vi "VolumeScanWizard 2.0.vi"(10 "Device order":i32[](array[numeric])=[0, 1], 11 "Device description":string[][](array[string])) -> (3 "Output":dbl[][](array[numeric]))   [LabVIEW 2015]
uses:
  <vilib>/gmath/NI_Gmath.lvlib
panel:
  in  "Cancel Button":bool
  in  "OK Button":bool
  in  "Ordering":u16(ring) items=["Raster", "Serpentine"]
  in  "Expression":string
  in  "Scan pattern":u16(ring) items=["Linear", "Exponential", "Logarithmic", "Quadratic", "Custom"]
  in  "Parameter table":string[][](table)
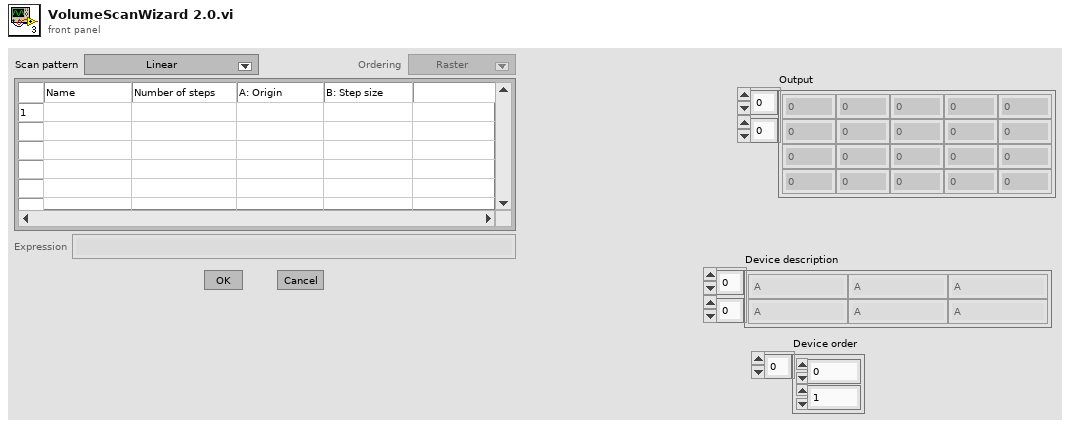
[diagram p1: front panel]
types:
  T1 = enum8{"Enabled", "Disabled", "Disabled and Grayed Out"}
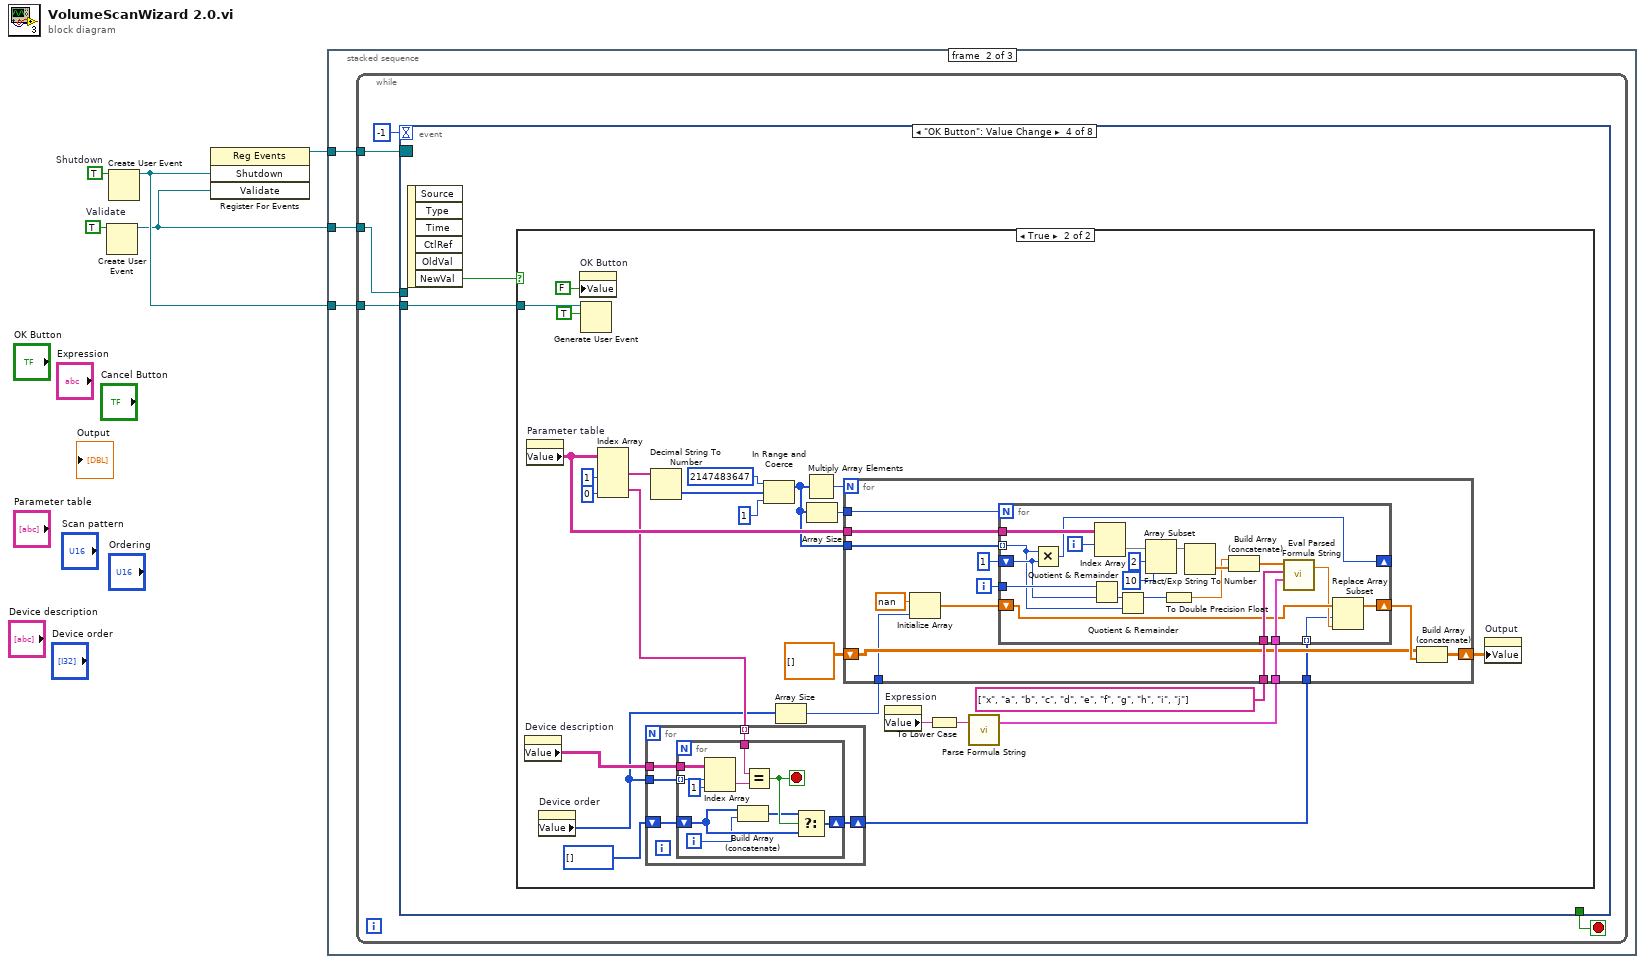
[diagram p0: block diagram]
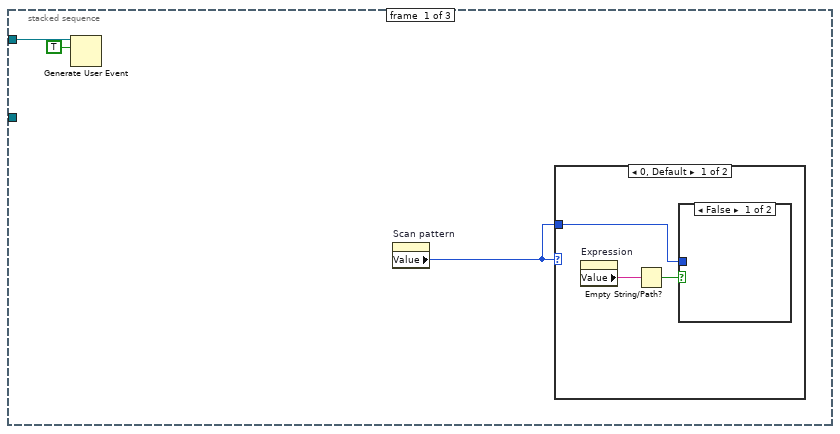
[diagram p2: hidden frame]
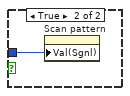
[diagram p3: hidden frame]
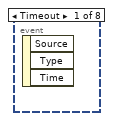
[diagram p5: hidden frame]
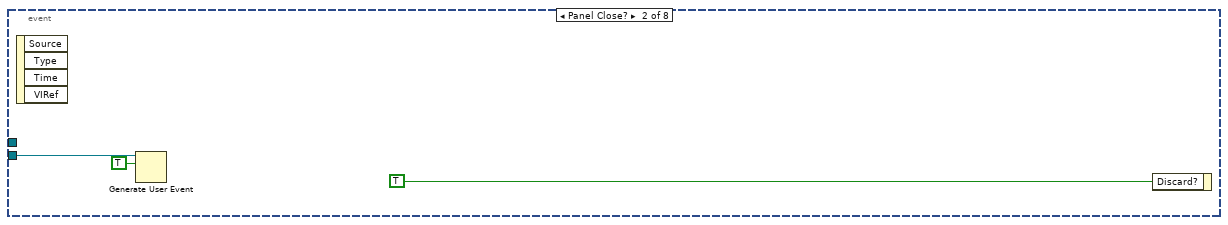
[diagram p6: hidden frame]
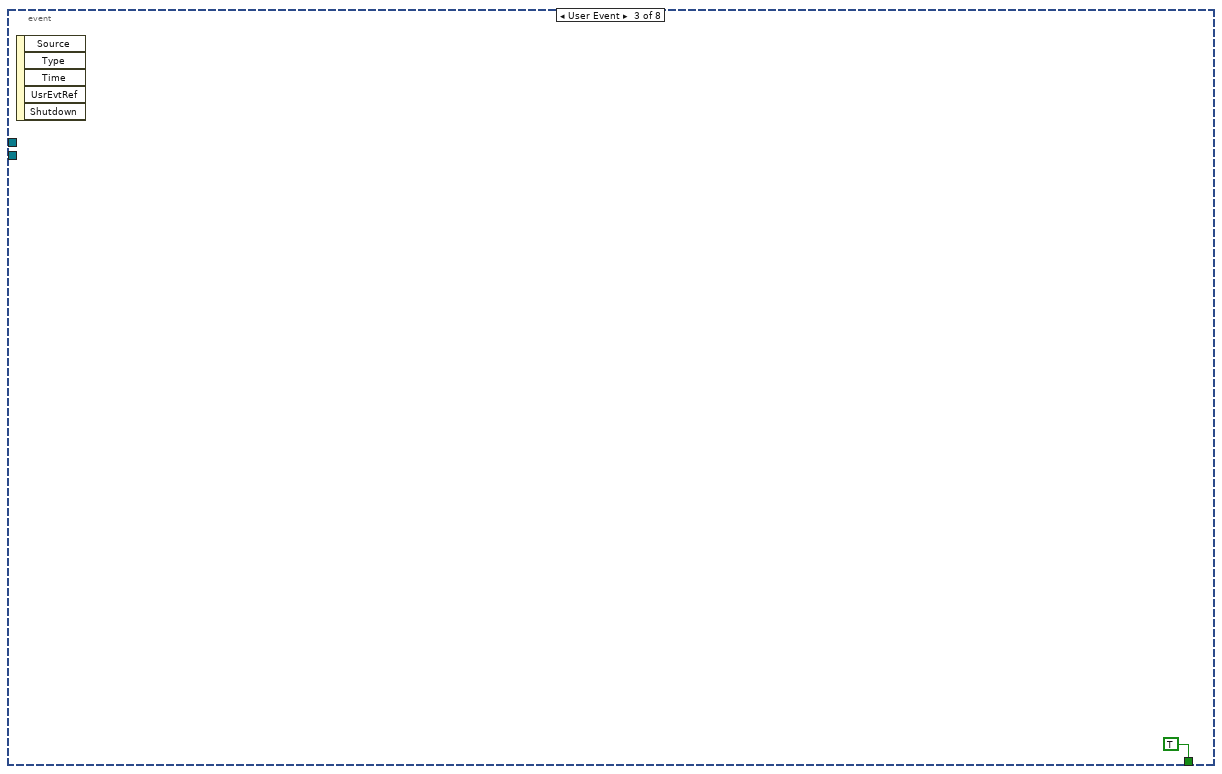
[diagram p7: hidden frame]
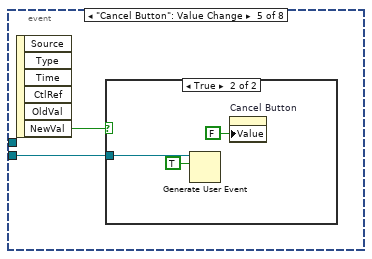
[diagram p9: hidden frame]
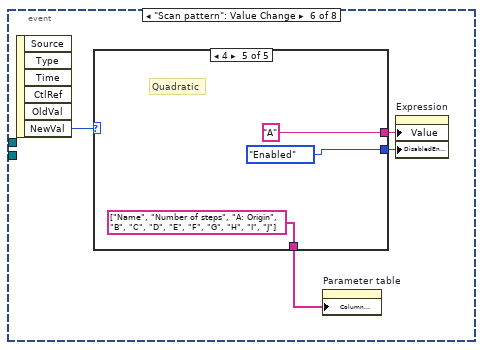
[diagram p11: hidden frame]
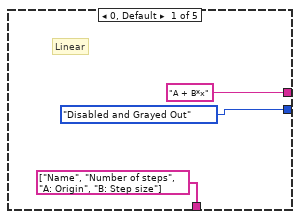
[diagram p12: hidden frame]
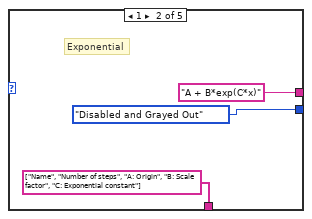
[diagram p13: hidden frame]
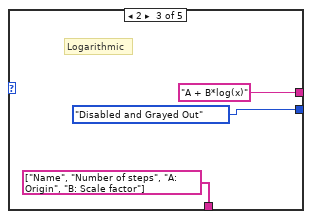
[diagram p14: hidden frame]
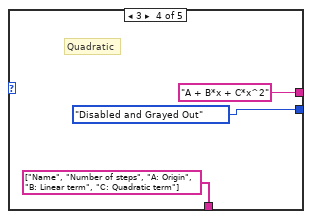
[diagram p15: hidden frame]
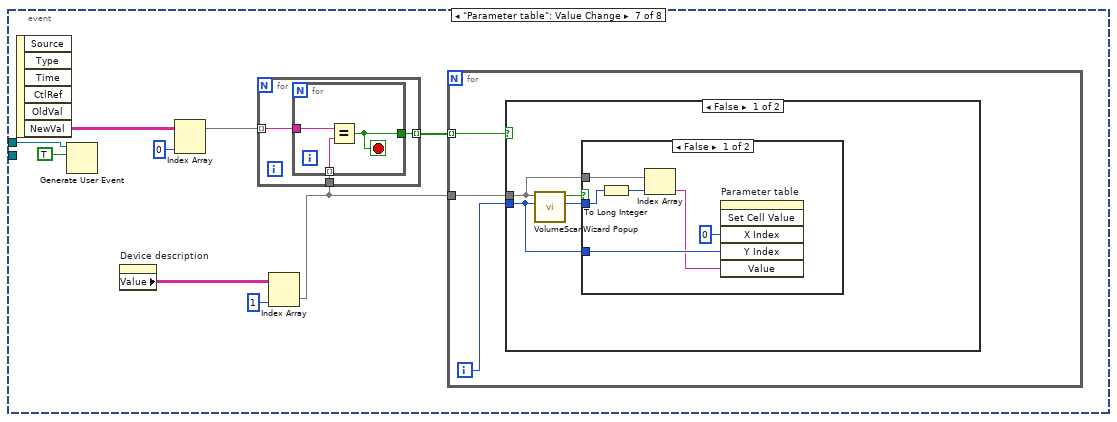
[diagram p16: hidden frame]
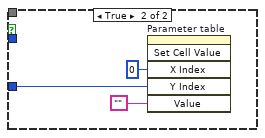
[diagram p17: hidden frame]
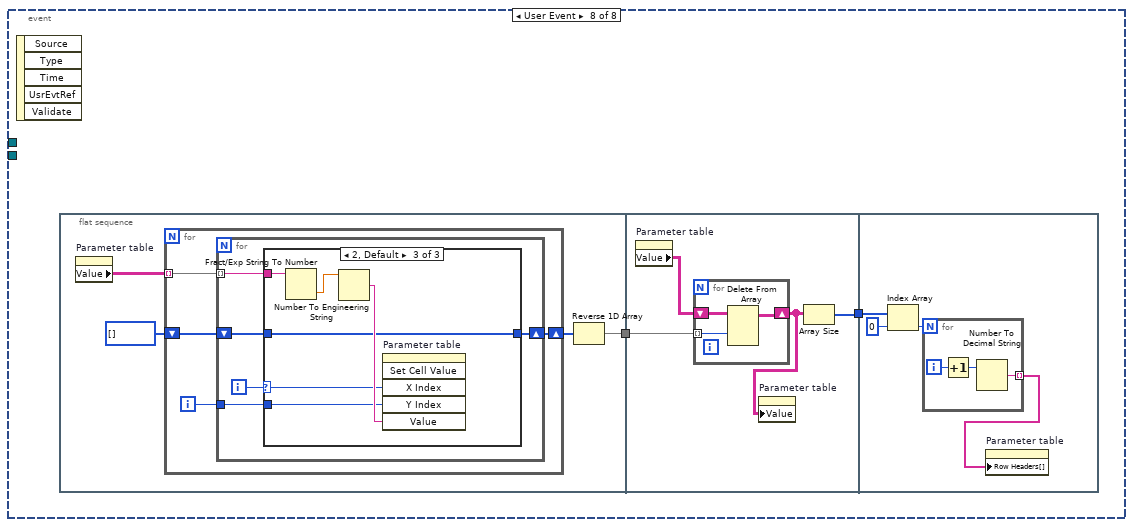
[diagram p19: hidden frame]
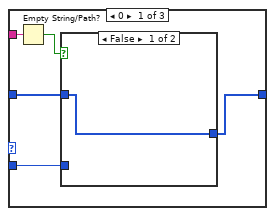
[diagram p20: hidden frame]
diagram:
  w2 = TRUE  # Validate
  w4 = TRUE  # Shutdown
  n1 = Create User Event(user event datatype=w2) -> (user event=w1:refnum<user-event>)  [unwired: 1 in, 1 out]
  n2 = Create User Event(user event datatype=w4) -> (user event=w3:refnum<user-event>)  [unwired: 1 in, 1 out]
  n3 = register-events(w3, w1) -> (reference out=w5:refnum<event-registration>)  [unwired: 2 in, 1 out]
  n4 = stacked-sequence {
    tunnel: w5 -> [_ w15 _]
    tunnel: w3 -> [_ w14 w207]
    tunnel: w1 -> [w8 w13 w208]
    frame #0 {
      n5 = Generate User Event(user event=w8, event data cluster=TRUE ("event data")) -> ()  [unwired: 2 in, 2 out]
      n6 = property on="Scan pattern" class="Ring (strict)"() -> ("Value"=w6:u16)  [unwired: 2 in, 2 out]
      n7 = case shown="0, Default" w6 {
        tunnel: w6 -> [w9 _]
        frame 0, Default {
          n8 = property on="Expression" class="Str"() -> ("Value"=w11:string)  [unwired: 2 in, 2 out]
          n9 = Empty String/Path?(string/path=w11) -> (empty?=w10:bool)
          n10 = case shown="False" w10 {
            tunnel: w9 -> [_ w12]
            frame False {
            }
            frame True {
              n11 = property on="Scan pattern" class="Ring (strict)"("Val(Sgnl)"=w12) -> ()  [unwired: 2 in, 2 out]
            }
          }
        }
        frame 4 {
        }
      }
    }
    frame #1 {
      n12 = while {
        tunnel: w15 -> [w19]
        tunnel: w14 -> [w17]
        tunnel: w13 -> [w16]
        stop <- w18 stop-if-true
        n13 = event shown="[3] \"OK Button\": Value Change" {
          selector: w19 -> [_ _ _ _ _ _ _ _]
          dyn-events: _ -> [_ _ _ _ _ _ _ _]
          timeout: -1 -> [_ _ _ _ _ _ _ _]
          tunnel: [_ _ TRUE _ _ _ _ _] -> w18
          tunnel: w17 -> [_ w22 _ w26 w103 _ _ _]
          tunnel: w16 -> [_ _ _ _ _ _ w134 _]
          event Timeout {
            n14 = event-data() -> ()  [unwired: 1 in, 3 out]
          }
          event Panel Close? {
            n15 = event-data() -> ()  [unwired: 1 in, 4 out]
            n16 = Generate User Event(user event=w22, event data cluster=TRUE ("event data")) -> ()  [unwired: 2 in, 2 out]
            n17 = event-data("Discard?"=TRUE) -> ()  [unwired: 1 in, 1 out]
          }
          event User Event {
            n18 = event-data() -> ()  [unwired: 1 in, 5 out]
          }
          event "OK Button": Value Change {
            n19 = event-data() -> ("NewVal"=w25:bool)  [unwired: 1 in, 5 out]
            n20 = case shown="True" w25 {
              tunnel: w26 -> [_ w51]
              frame False {
              }
              frame True {
                n21 = property on="Device description" class="Arr (strict)"() -> ("Value"=w32:string[][])  [unwired: 2 in, 2 out]
                n22 = property on="Parameter table" class="Tbl (strict)"() -> ("Value"=w41:string[][])  [unwired: 2 in, 2 out]
                n23 = property on="Device order" class="Arr (strict)"() -> ("Value"=w27:i32[])  [unwired: 2 in, 2 out]
                n24 = property on="OK Button" class="Bool (strict)"("Value"=FALSE ("OK Button")) -> ()  [unwired: 2 in, 2 out]
                n25 = Generate User Event(user event=w51, event data cluster=TRUE ("event data")) -> ()  [unwired: 2 in, 2 out]
                n26 = Index Array(array=w41, index (col) #1=1 ("disabled index (col)"), index (col) #2=0 ("index (col)")) -> (element #1=w47:string[], element #2=w31:string[])  [unwired: 2 in]
                n27 = for {
                  tunnel: w32 -> [w56]
                  tunnel: w27 -> [w55]
                  tunnel: w31 -> [w54] mode=indexing
                  shift-right: [w52] -> w29
                  shift-left: i32[] [] -> [w53]
                  n28 = for {
                    tunnel: w56 -> [w66]
                    tunnel: w55 -> [w65] mode=indexing
                    tunnel: w54 -> [w63]
                    shift-right: [w61] -> w52
                    shift-left: w53 -> [w60]
                    i -> [w57]
                    stop <- w62 stop-if-true
                    n29 = Index Array(array=w66, index (row)=w65, index (col)=1 ("disabled index (col)")) -> (element=w58:string)
                    n30 = Build Array (concatenate)(w60, w57) -> (w59:i32[])
                    n31 = Equal?(x=w63, y=w58) -> (x = y?=w62:bool)
                    n32 = Select(t=w59, s=w62, f=w60) -> (s? t:f=w61:i32[])
                  }
                }
                n33 = Decimal String To Number(string=w47) -> (number=w46:i32[])  [unwired: 2 in, 1 out]
                n34 = In Range and Coerce(upper limit=2147483647, x=w46, lower limit=1) -> (coerced(x)=w38:i32[])  [unwired: 1 out]
                n35 = Array Size(array=w27) -> (size(s)=w28:i32)
                n36 = Multiply Array Elements(1:w38) -> (0:w44:i32)
                n37 = Array Size(array=w38) -> (size(s)=w43:i32)
                n38 = property on="Expression" class="Str"() -> ("Value"=w35:string)  [unwired: 2 in, 2 out]
                n39 = To Lower Case(string=w35) -> (all lower case string=w34:string)
                n40 = call <vilib>:"Parse Formula String.vi"("formula"=w34) -> ("Parsed Formula"=w40:cluster{"Table":i32[][], "Y Values":dbl[]})  [unwired: 1 in, 1 out]
                n41 = for {
                  N: w44 -> [_]
                  tunnel: w43 -> [w78]
                  tunnel: w41 -> [w80]
                  tunnel: w40 -> [w76]
                  tunnel: string[] ["x", "a", "b", "c", "d", "e", "f", "g", "h", "i", "j"] ("Variables") -> [w75]
                  tunnel: w38 -> [w70]
                  shift-right: [w71] -> w36
                  shift-left: dbl[][] [] -> [w72]
                  tunnel: w29 -> [w68]
                  tunnel: w28 -> [w67]
                  i -> [w74]
                  n42 = Initialize Array(nan ("element"), w67) -> (w79:dbl[])
                  n43 = for {
                    N: w78 -> [_]
                    tunnel: w80 -> [w101]
                    shift-right: [w89] -> w73
                    shift-left: w79 -> [w88]
                    tunnel: w76 -> [w97]
                    tunnel: w75 -> [w96]
                    tunnel: w74 -> [w85]
                    shift-right: [w92] -> _
                    shift-left: 1 -> [w83]
                    tunnel: w70 -> [w82] mode=indexing
                    tunnel: w68 -> [w81] mode=indexing
                    i -> [w86]
                    n44 = Multiply(x=w82, y=w83) -> (x*y=w92:i32)
                    n45 = Quotient & Remainder(x=w85, y=w83) -> (floor(x/y)=w84:i32)  [unwired: 1 out]
                    n46 = Index Array(array=w101, index (row)=w86) -> (element=w100:string[])  [unwired: 1 in]
                    n47 = Quotient & Remainder(x=w84, y=w82) -> (x-y*floor(x/y)=w91:i32)  [unwired: 1 out]
                    n48 = Array Subset(array=w100, index=2, length=10) -> (w99:string[])
                    n49 = To Double Precision Float(number=w91) -> (double precision float=w90:dbl)
                    n50 = Fract/Exp String To Number(string=w99) -> (number=w95:dbl[])  [unwired: 3 in, 1 out]
                    n51 = Build Array (concatenate)(w90, w95) -> (w94:dbl[])
                    n52 = call <vilib>:"Eval Parsed Formula String.vi"("Parsed Formula"=w97, "Variables"=w96, "X Values"=w94) -> ("y value"=w87:dbl)  [unwired: 1 in, 1 out]
                    n53 = Replace Array Subset(array=w88, new element=w87, index=w81) -> (w89:dbl[])
                  }
                  n54 = Build Array (concatenate)(w72, w73) -> (w71:dbl[][])
                }
                n55 = property on="Output" class="Arr (strict)"("Value"=w36) -> ()  [unwired: 2 in, 2 out]
              }
            }
          }
          event "Cancel Button": Value Change {
            n56 = event-data() -> ("NewVal"=w102:bool)  [unwired: 1 in, 5 out]
            n57 = case shown="True" w102 {
              tunnel: w103 -> [_ w106]
              frame False {
              }
              frame True {
                n58 = Generate User Event(user event=w106, event data cluster=TRUE ("event data")) -> ()  [unwired: 2 in, 2 out]
                n59 = property on="Cancel Button" class="Bool (strict)"("Value"=FALSE ("Cancel Button")) -> ()  [unwired: 2 in, 2 out]
              }
            }
          }
          event "Scan pattern": Value Change {
            n60 = event-data() -> ("NewVal"=w110:u16)  [unwired: 1 in, 5 out]
            n61 = case shown="4" w110 {
              tunnel: ["A + B*x" "A + B*exp(C*x)" "A + B*log(x)" "A + B*x + C*x^2" "A"] -> w109
              tunnel: [T1."Disabled and Grayed Out" ("Disabled") T1."Disabled and Grayed Out" ("Disabled") T1."Disabled and Grayed Out" ("Disabled") T1."Disabled and Grayed Out" ("Disabled") T1."Enabled" ("Disabled")] -> w108
              tunnel: [string[] ["Name", "Number of steps", "A: Origin", "B: Step size"] ("Column Header Strings[]") string[] ["Name", "Number of steps", "A: Origin", "B: Scale factor", "C: Exponential constant"] ("Column Header Strings[]") string[] ["Name", "Number of steps", "A: Origin", "B: Scale factor"] ("Column Header Strings[]") string[] ["Name", "Number of steps", "A: Origin", "B: Linear term", "C: Quadratic term"] ("Column Header Strings[]") string[] ["Name", "Number of steps", "A: Origin", "B", "C", "D", "E", "F", "G", "H", "I", "J"] ("Column Header Strings[]")] -> w107
              frame 0, Default {
                # "Linear"
              }
              frame 1 {
                # "Exponential"
              }
              frame 2 {
                # "Logarithmic"
              }
              frame 3 {
                # "Quadratic"
              }
              frame 4 {
                # "Quadratic"
              }
            }
            n62 = property on="Parameter table" class="Tbl (strict)"("Column Headers[]"=w107) -> ()  [unwired: 2 in, 2 out]
            n63 = property on="Expression" class="Str"("Value"=w109, "DisabledEnum"=w108) -> ()  [unwired: 2 in, 2 out]
          }
          event "Parameter table": Value Change {
            n64 = event-data() -> ("NewVal"=w130:string[][])  [unwired: 1 in, 5 out]
            n65 = Generate User Event(user event=w134, event data cluster=TRUE ("event data")) -> ()  [unwired: 2 in, 2 out]
            n66 = property on="Device description" class="Arr (strict)"() -> ("Value"=w132:string[][])  [unwired: 2 in, 2 out]
            n67 = Index Array(array=w130, index (col)=0 ("disabled index (col)")) -> (element=w129:string[])  [unwired: 1 in]
            n68 = Index Array(array=w132, index (col)=1 ("disabled index (col)")) -> (element=w127:string[])  [unwired: 1 in]
            n69 = for {
              tunnel: w129 -> [w137] mode=indexing
              tunnel: w127 -> [w136]
              tunnel: [w135] -> w126 mode=indexing
              n70 = for {
                tunnel: w137 -> [w139]
                tunnel: w136 -> [w140] mode=indexing
                tunnel: [w138] -> w135
                stop <- w138 stop-if-true
                n71 = Equal?(x=w139, y=w140) -> (x = y?=w138:bool)
              }
            }
            n72 = for {
              tunnel: w126 -> [w143] mode=indexing
              tunnel: w127 -> [w141]
              i -> [w142]
              n73 = case shown="False" w143 {
                tunnel: w142 -> [w146 _]
                tunnel: w141 -> [w144 _]
                frame False {
                  n74 = call "VolumeScanWizard Popup.vi"("Row"=w146, "Axes"=w144) -> ("Selection"=w145:u16, "Cancelled"=w147:bool)  [unwired: 8 in]
                  n75 = case shown="False" w147 {
                    tunnel: w146 -> [w153 w156]
                    tunnel: w145 -> [w150 _]
                    tunnel: w144 -> [w151 _]
                    frame False {
                      n76 = To Long Integer(number=w150) -> (32bit integer=w148:i32)
                      n77 = Index Array(array=w151, index=w148) -> (element=w149:string)
                      n78 = invoke on="Parameter table" class="Tbl (strict)" method="Set Cell Value"("X Index"=0, "Y Index"=w153, "Value"=w149) -> ()  [unwired: 3 in, 6 out]
                    }
                    frame True {
                      n79 = invoke on="Parameter table" class="Tbl (strict)" method="Set Cell Value"("X Index"=0, "Y Index"=w156, "Value"="") -> ()  [unwired: 3 in, 6 out]
                    }
                  }
                }
                frame True {
                }
              }
            }
          }
          event User Event {
            n80 = event-data() -> ()  [unwired: 1 in, 5 out]
            n81 = flat-sequence {
              tunnel: [w161] -> w158
              tunnel: w158 -> [w196]
              tunnel: [w193] -> w157
              tunnel: w157 -> [w203]
              frame #0 {
                n82 = property on="Parameter table" class="Tbl (strict)"() -> ("Value"=w160:string[][])  [unwired: 2 in, 2 out]
                n83 = for {
                  tunnel: w160 -> [w166] mode=indexing
                  shift-right: [w164] -> w162
                  shift-left: i32[] [] -> [w163]
                  i -> [w165]
                  n84 = for {
                    tunnel: w166 -> [w170] mode=indexing
                    tunnel: w165 -> [w169]
                    shift-right: [w168] -> w164
                    shift-left: w163 -> [w167]
                    i -> [w171]
                    n85 = case shown="2, Default" w171 {
                      selector: w171 -> [_ w184 w191]
                      tunnel: w170 -> [w176 w182 w189]
                      tunnel: w169 -> [w174 w183 w190]
                      tunnel: [w173 w181 w187] -> w168
                      tunnel: w167 -> [w172 w181 w187]
                      frame 0 {
                        n86 = Empty String/Path?(string/path=w176) -> (empty?=w175:bool)
                        n87 = case shown="False" w175 {
                          tunnel: w174 -> [_ w180]
                          tunnel: [w177 w179] -> w173
                          tunnel: w172 -> [w177 w178]
                          frame False {
                          }
                          frame True {
                            n88 = Build Array (concatenate)(w178, w180) -> (w179:i32[])
                          }
                        }
                      }
                      frame 1 {
                        n89 = Decimal String To Number(string=w182) -> (number=w185:i32)  [unwired: 2 in, 1 out]
                        n90 = Number To Decimal String(number=w185) -> (decimal integer string=w186:string)  [unwired: 1 in]
                        n91 = invoke on="Parameter table" class="Tbl (strict)" method="Set Cell Value"("X Index"=w184, "Y Index"=w183, "Value"=w186) -> ()  [unwired: 3 in, 6 out]
                      }
                      frame 2, Default {
                        n92 = Fract/Exp String To Number(string=w189) -> (number=w188:dbl)  [unwired: 3 in, 1 out]
                        n93 = Number To Engineering String(4:w188) -> (0:w192:string)  [unwired: 3 in]
                        n94 = invoke on="Parameter table" class="Tbl (strict)" method="Set Cell Value"("X Index"=w191, "Y Index"=w190, "Value"=w192) -> ()  [unwired: 3 in, 6 out]
                      }
                    }
                  }
                }
                n95 = Reverse 1D Array(array=w162) -> (reversed array=w161:i32[])
              }
              frame #1 {
                n96 = property on="Parameter table" class="Tbl (strict)"() -> ("Value"=w195:string[][])  [unwired: 2 in, 2 out]
                n97 = for {
                  tunnel: w196 -> [w199] mode=indexing
                  shift-right: [w197] -> w194
                  shift-left: w195 -> [w198]
                  n98 = Delete From Array(array=w198, index (row)=w199) -> (array with subset deleted=w197:string[][])  [unwired: 2 in, 1 out]
                }
                n99 = property on="Parameter table" class="Tbl (strict)"("Value"=w194) -> ()  [unwired: 2 in, 2 out]
                n100 = Array Size(array=w194) -> (size(s)=w193:i32[])
              }
              frame #2 {
                n101 = Index Array(array=w203, index=0) -> (element=w201:i32)
                n102 = for {
                  N: w201 -> [_]
                  tunnel: [w205] -> w200 mode=indexing
                  i -> [w206]
                  n103 = Increment(x=w206) -> (x+1=w204:i32)
                  n104 = Number To Decimal String(number=w204) -> (decimal integer string=w205:string)  [unwired: 1 in]
                }
                n105 = property on="Parameter table" class="Tbl (strict)"("Row Headers[]"=w200) -> ()  [unwired: 2 in, 2 out]
              }
            }
          }
        }
      }
    }
    frame #2 {
      n106 = Destroy User Event(user event=w207) -> ()  [unwired: 1 in, 1 out]
      n107 = Destroy User Event(user event=w208) -> ()  [unwired: 1 in, 1 out]
    }
  }
